vi "Check Cursor Status.vi"(7 "Cursor Property Array In":T1, 8 "error in (no error)":errorcluster, 9 "Coords":cluster{"Horizontal":i32, "Vertical":i32}, 11 "3D Picture Control In":refnum<vi>) -> (0 "error out":errorcluster, 1 "Drag Cursor?":bool, 2 "Cursor ID":i32, 3 "3D Picture Control Out":refnum<vi>, 5 "Cursor Property Array Out":T1)   [LabVIEW 2020, in "3D Plot.lvclass"]
uses:
  <vilib>/Math Plots/3D Math Plots/3D Plot/3D Plot/3D Plot.lvclass
  <vilib>/Math Plots/3D Math Plots/3D Plot/3D Plot/Typedef/Cursor Property Array.ctl
  <vilib>/Math Plots/3D Math Plots/3D Plot/3D Plot/Typedef/Cursor Property.ctl
  <vilib>/Math Plots/3D Math Plots/3D Plot/3D Plot/Typedef/Cursor Position.ctl
  <vilib>/Math Plots/3D Math Plots/3D Plot/3D Plot/Typedef/Cursor Point.ctl
  <vilib>/Math Plots/3D Math Plots/3D Plot/3D Plot/Typedef/Sprite Type.ctl
  <vilib>/Math Plots/3D Math Plots/3D Plot/3D Plot/Typedef/Cursor Line.ctl
  <vilib>/Math Plots/3D Math Plots/3D Plot/3D Plot/Typedef/Line Type.ctl
  <vilib>/Math Plots/3D Math Plots/3D Plot/3D Plot/Typedef/Cursor Plane.ctl
  <vilib>/Math Plots/3D Math Plots/3D Plot/3D Plot/Typedef/Cursor Text.ctl
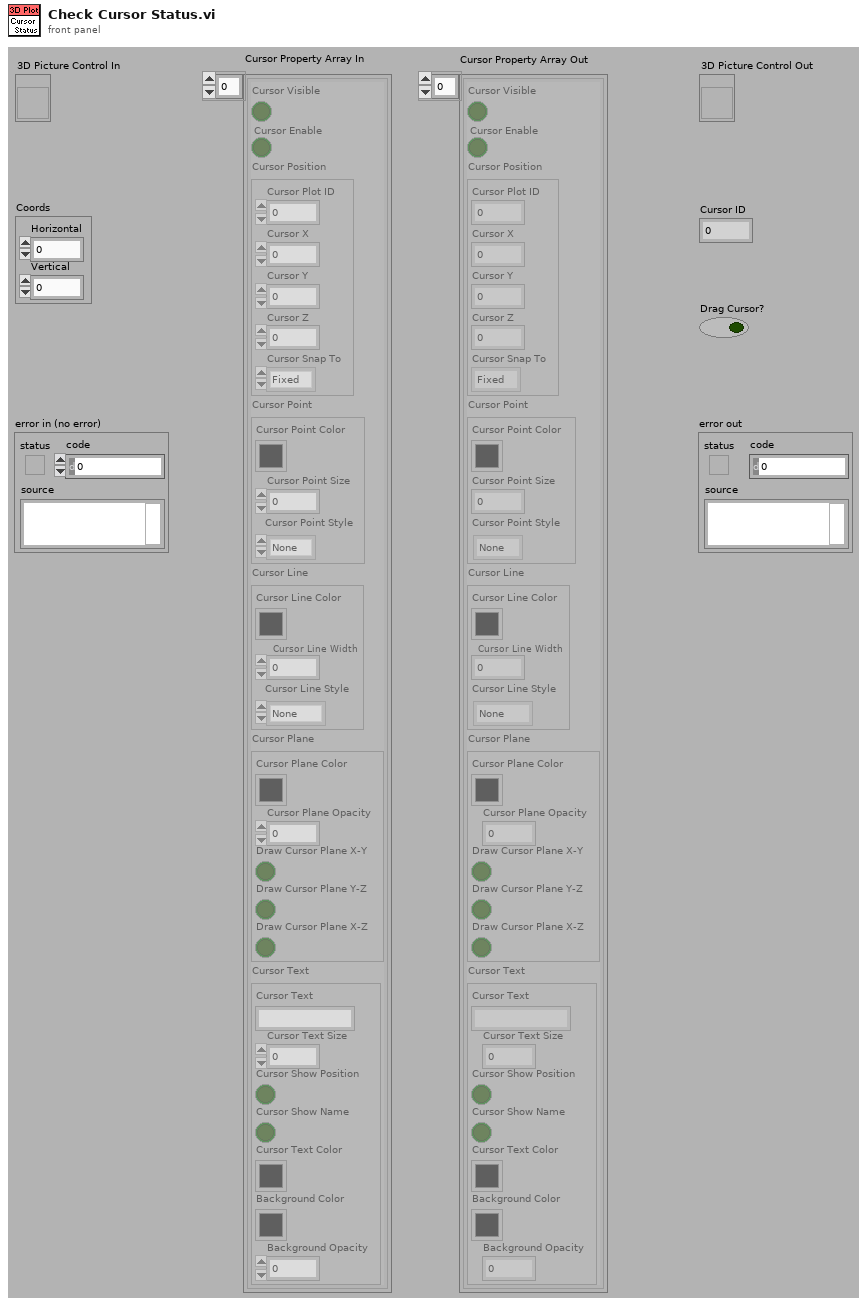
[diagram p1: front panel]
types:
  T1 = typedef "3D Plot.lvclass/Cursor Property Array.ctl" = T2[]
  T2 = typedef "3D Plot.lvclass/Cursor Property.ctl" = cluster{"Cursor Visible":bool, "Cursor Enable":bool, "Cursor Position":T3, "Cursor Point":T4, "Cursor Line":T6, "Cursor Plane":T8, "Cursor Text":T9}
  T3 = typedef "3D Plot.lvclass/Cursor Position.ctl" = cluster{"Cursor Plot ID":i32, "Cursor X":sgl, "Cursor Y":sgl, "Cursor Z":sgl, "Cursor Snap To":enum16{"Fixed", "Nearest Plot", "Snap to Plot"}}
  T4 = typedef "3D Plot.lvclass/Cursor Point.ctl" = cluster{"Cursor Point Color":u32, "Cursor Point Size":sgl, "Cursor Point Style":T5}
  T5 = typedef "3D Plot.lvclass/Sprite Type.ctl" = enum16{"None", "Empty Square", "Solid Square", "Empty Diamond", "Solid Diamond", "Empty Circle", "Solid Circle", "Asterisk", "Bold X", "Wireframe Sphere", "Solid Sphere", "Wireframe Cube", "Solid Cube"}
  T6 = typedef "3D Plot.lvclass/Cursor Line.ctl" = cluster{"Cursor Line Color":u32, "Cursor Line Width":sgl, "Cursor Line Style":T7}
  T7 = typedef "3D Plot.lvclass/Line Type.ctl" = enum16{"None", "Solid", "Dash", "Dot", "Dash Dot"}
  T8 = typedef "3D Plot.lvclass/Cursor Plane.ctl" = cluster{"Cursor Plane Color":u32, "Cursor Plane Opacity":sgl, "Draw Cursor Plane X-Z":bool, "Draw Cursor Plane Y-Z":bool, "Draw Cursor Plane X-Y":bool}
  T9 = typedef "3D Plot.lvclass/Cursor Text.ctl" = cluster{"Cursor Text":string, "Cursor Text Size":u16, "Cursor Show Position":bool, "Cursor Show Name":bool, "Cursor Text Color":u32, "Background Color":u32, "Background Opacity":sgl}
  T10 = typedef "LVPoint32TypeDef.ctl" = cluster{"Horizontal":i32, "Vertical":i32}
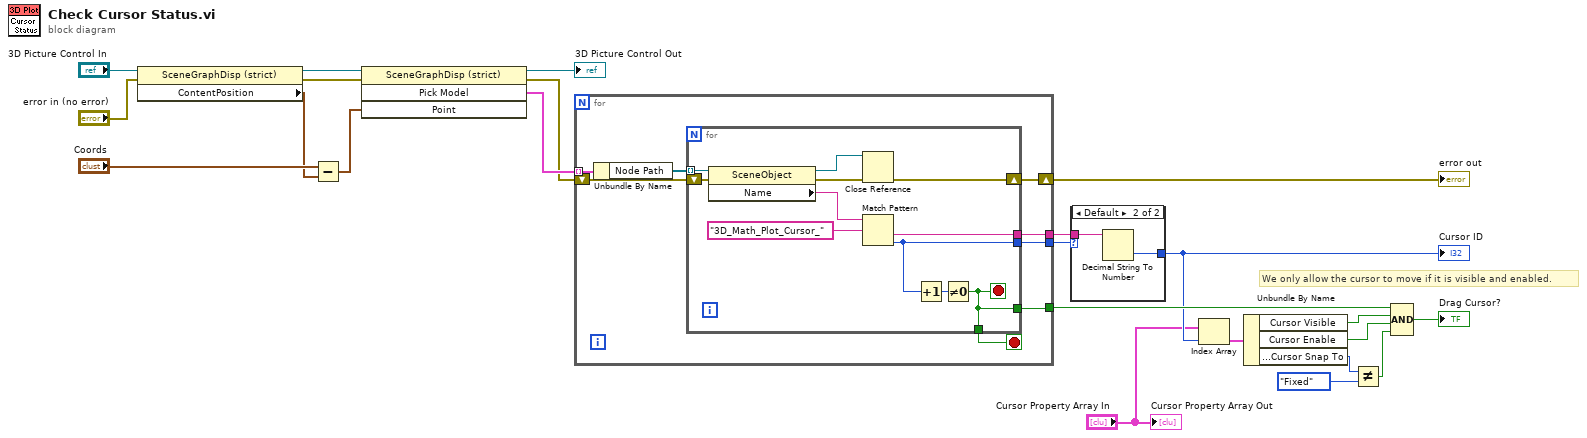
[diagram p0: block diagram]
diagram:
  # "We only allow the cursor to move if it is visible and enabled."
  n1 = property class="SceneGraphDisp (strict)"(reference="3D Picture Control In", error in="error in (no error)") -> (reference out=w15:refnum<vi>, error out=w14:errorcluster, "ContentPosition"=w16:T10)
  n2 = Subtract(x="Coords", y=w16) -> (x-y=w13:T10)
  n3 = invoke class="SceneGraphDisp (strict)" method="Pick Model"(reference=w15, error in=w14, "Point"=w13) -> (reference out=→"3D Picture Control Out":refnum<vi>, error out=w11:errorcluster, "Pick Model"=w12:cluster{"Node Path":refnum<vi>[]}[])  [unwired: 1 in, 1 out]
  n4 = for {
    tunnel: w12 -> [w31] mode=indexing
    shift-right: [w28] -> w6
    shift-left: w11 -> [w29]
    tunnel: [w26] -> w10
    tunnel: [w25] -> w9
    tunnel: [w24] -> w4
    stop <- w27 stop-if-true
    n5 = Unbundle By Name(w31) -> ("Node Path"=w30:refnum<vi>[])
    n6 = for {
      tunnel: w30 -> [w42] mode=indexing
      shift-right: [w32] -> w28
      shift-left: w29 -> [w41]
      tunnel: [w37] -> w27
      tunnel: [w37] -> w26
      tunnel: [w36] -> w25
      tunnel: [w35] -> w24
      stop <- w37 stop-if-true
      n7 = property class="SceneObject"(reference=w42, error in=w41) -> (reference out=w34:refnum<vi>, error out=w33:errorcluster, "Name"=w40:string)
      n8 = Close Reference(reference=w34, error in (no error)=w33) -> (error out=w32:errorcluster)
      n9 = Match Pattern(string=w40, regular expression="3D_Math_Plot_Cursor_" ("string")) -> (after substring=w36:string, offset past match=w35:i32)  [unwired: 3 out]
      n10 = Increment(x=w35) -> (x+1=w38:i32)
      n11 = Not Equal To 0?(x=w38) -> (x != 0?=w37:bool)
    }
  }
  "error out" <- w6
  n12 = case shown="Default" w4 {
    selector: w4 -> [w43 _]
    tunnel: w9 -> [_ w45]
    tunnel: [w43 w44] -> w8
    frame -1 {
    }
    frame Default {
      n13 = Decimal String To Number(string=w45) -> (number=w44:i32)  [unwired: 3 out]
    }
  }
  "Cursor ID" <- w8
  n14 = Index Array(array="Cursor Property Array In", index=w8) -> (element=w20:T2)
  n15 = Unbundle By Name(w20) -> ("Cursor Visible"=w22:bool, "Cursor Enable"=w21:bool, "Cursor Position.Cursor Snap To"=w3:enum16{"Fixed", "Nearest Plot", "Snap to Plot"})
  n16 = Not Equal?(x=w3, y=enum16{"Fixed", "Nearest Plot", "Snap to Plot"}."Fixed" ("Cursor Position.Cursor Snap To")) -> (x != y?=w1:bool)
  n17 = Compound Arithmetic op=AND(w10, w22, w21, w1) -> (→"Drag Cursor?":bool)
  "Cursor Property Array Out" <- "Cursor Property Array In"
